vi "Cluster to Element Details.vi"(8 "error in":errorcluster, 11 "Cluster":variant) -> (0 "error out":errorcluster, 1 "gRPC Enum Metadata":T1[](array[typedef]), 2 "More Cluster":variant[](array[variant]), 3 "gRPC Message Metadata":T2)   [LabVIEW 2019, in "grpc-lvsupport.lvlib"]
uses:
  grpc-lvsupport.lvlib
  typeDefs/Message Metadata.ctl
  typeDefs/Message Element Metadata.ctl
  typeDefs/Message Element Type.ctl
  typeDefs/Enum Metadata.ctl
  <vilib>/Utility/Data Type/NI_Data Type.lvlib
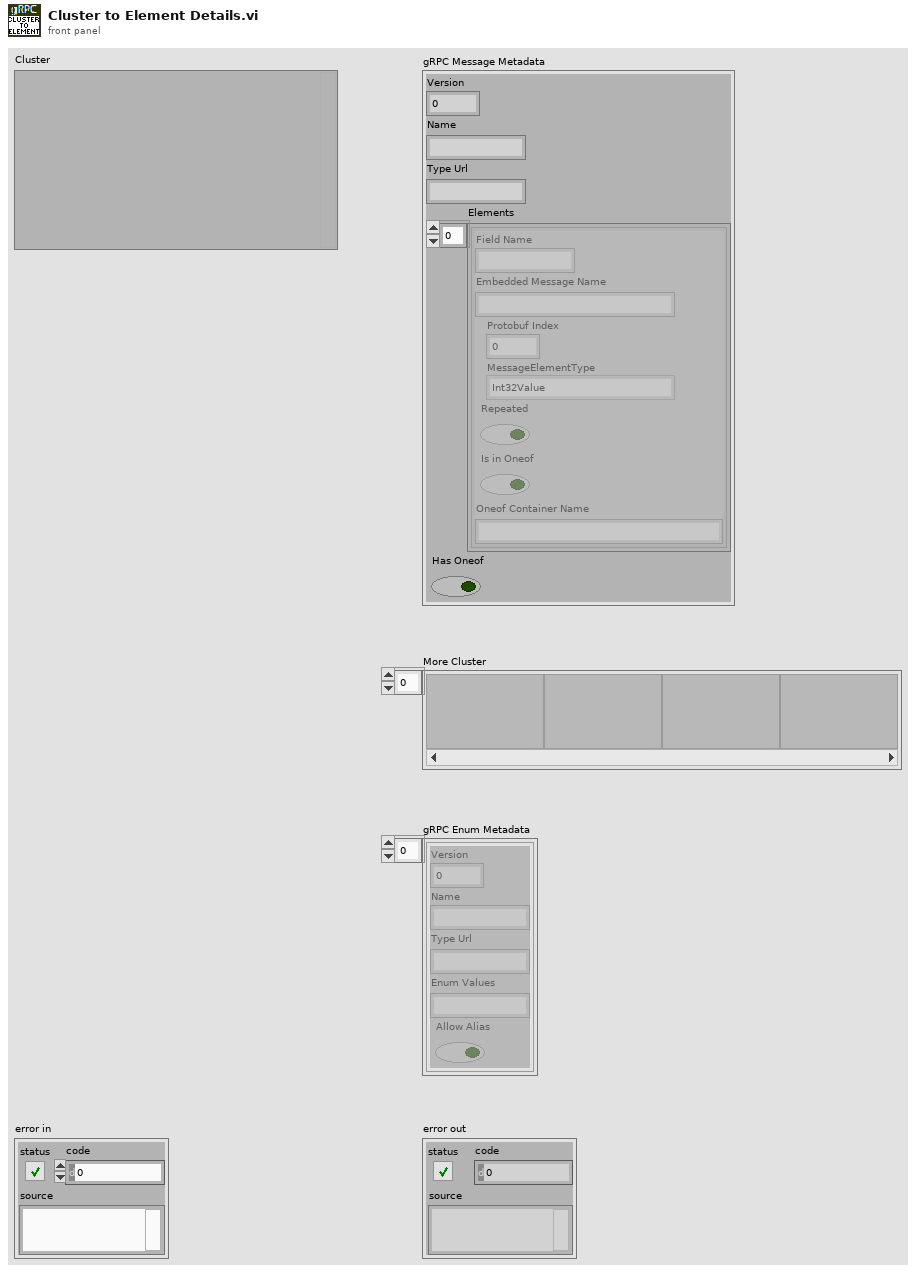
[diagram p1: front panel]
types:
  T1 = typedef "grpc-lvsupport.lvlib/Enum Metadata.ctl" = cluster{"Version":i32, "Name":string, "Type Url":string, "Enum Values":string, "Allow Alias":bool}
  T2 = typedef "grpc-lvsupport.lvlib/Message Metadata.ctl" = cluster{"Version":i32, "Name":string, "Type Url":string, "Elements":T3[], "Has Oneof":bool}
  T3 = typedef "grpc-lvsupport.lvlib/Message Element Metadata.ctl" = cluster{"Field Name":string, "Embedded Message Name":string, "Protobuf Index":i32, "MessageElementType":T4, "Repeated":bool, "Is in Oneof":bool, "Oneof Container Name":string}
  T4 = typedef "grpc-lvsupport.lvlib/Message Element Type.ctl" = enum32{"Int32Value", "FloatValue", "DoubleValue", "BoolValue", "StringValue", "MessageValue", "Int64Value", "UInt32Value", "UInt64Value", "EnumValue", "Bytes", "Fixed64", "Fixed32", "SFixed64", "SFixed32", "SInt64", "SInt32"}
  T5 = typedef "NI_Data Type.lvlib/Data Type.ctl" = enum8{"Invalid Type", "Void", "I8", "I16", "I32", "I64", "U8", "U16", "U32", "U64", "Single Float", "Double Float", "Extended Float", "Single Complex", "Double Complex", "Extended Complex", "Enum U8", "Enum U16", "Enum U32", "Enum U64", "Single Float With Unit", "Double Float With Unit", "Extended Float With Unit", "Single Complex with Unit", "Double Complex with Unit", "Extended Complex with Unit", "Boolean", "String", "Path", "Picture", "Tag", "Array", "Cluster", "Variant", "LV Variant", "Waveform", "Timestamp", "Digital Waveform", "Digital Data", "ExpressData", "Refnum", "External Data", "VI", "Poly VI", "LabVIEW Class Instance", "Fixed Point", "Set Collection", "Map Collection"}
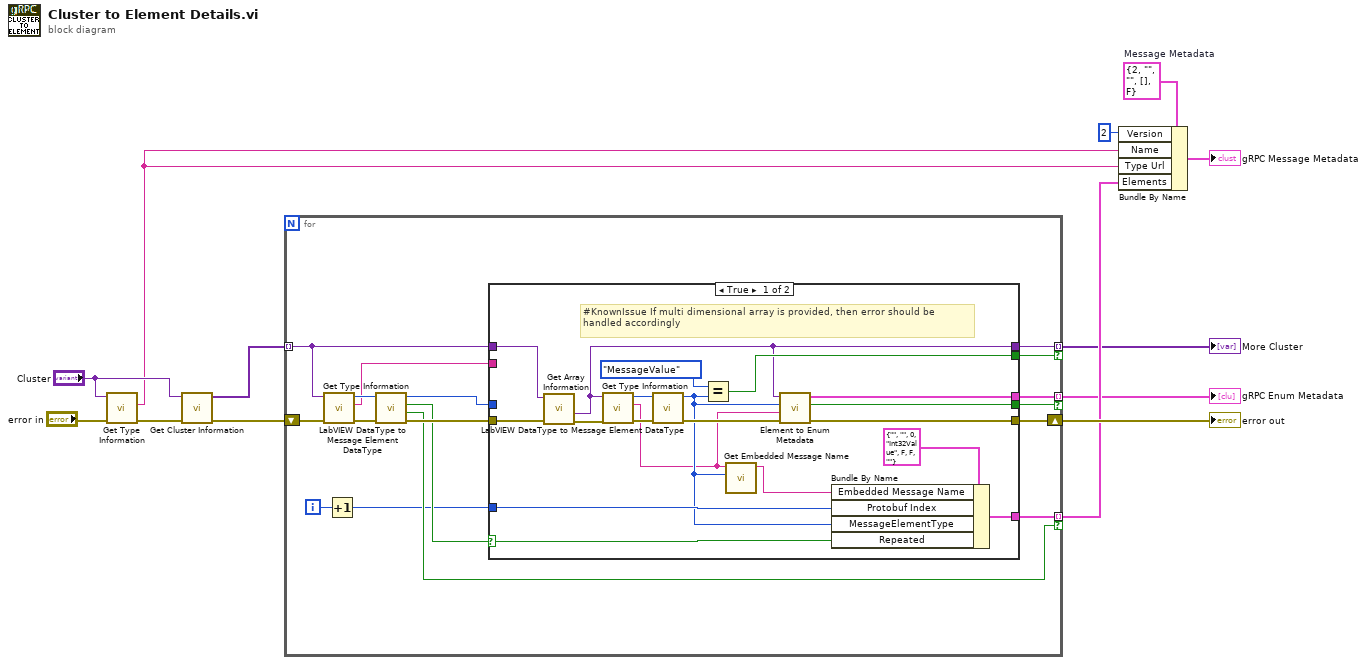
[diagram p0: block diagram]
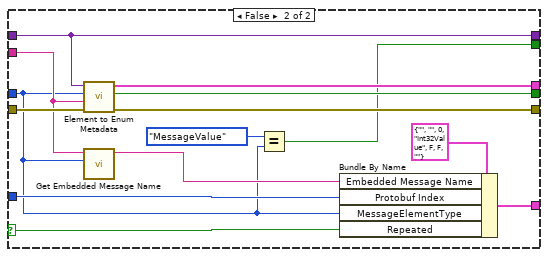
[diagram p2: hidden frame]
diagram:
  w9 = T2 {"Version"=2, "Name"="", "Type Url"="", "Elements"=[], "Has Oneof"=FALSE}  # Message Metadata
  n1 = call <vilib>:"Get Type Information.vi"("error in (no error)"="error in", "variant"="Cluster") -> ("error out"=w13:errorcluster, "name"=w5:string)  [unwired: 5 in, 3 out]
  n2 = call <vilib>:"Get Cluster Information.vi"("error in (no error)"=w13, "variant"="Cluster") -> ("error out"=w12:errorcluster, "cluster elements"=w6:variant[])  [unwired: 8 in]
  n3 = for {
    tunnel: w6 -> [w21] mode=indexing
    tunnel: [w23] -> w4 mode=indexing if=w22
    shift-right: [w27] -> w11
    shift-left: w12 -> [w30]
    tunnel: [w18] -> w3 mode=indexing if=w17
    tunnel: [w15] -> w1 mode=indexing if=w14
    i -> [w26]
    n4 = call <vilib>:"Get Type Information.vi"("error in (no error)"=w30, "variant"=w21) -> ("error out"=w29:errorcluster, "name"=w19:string, "type"=w25:T5)  [unwired: 5 in, 2 out]
    n5 = Increment(x=w26) -> (x+1=w20:i32)
    n6 = call "LabVIEW DataType to Message Element DataType.vi"("error in"=w29, "type"=w25) -> ("error out"=w28:errorcluster, "Supported?"=w22:bool, "Array?"=w24:bool, "MessageElementType"=w16:T4)  [unwired: 6 in]
    n7 = case shown="True" w24 {
      selector: w24 -> [w44 w61]
      tunnel: w20 -> [w46 w63]
      tunnel: [w43 w60] -> w23
      tunnel: w28 -> [w49 w59]
      tunnel: w21 -> [w42 w58]
      tunnel: [w36 w57] -> w27
      tunnel: w19 -> [_ w54]
      tunnel: [w33 w58] -> w18
      tunnel: [w39 w50] -> w17
      tunnel: w16 -> [_ w52]
      tunnel: [w34 w56] -> w15
      tunnel: [w35 w55] -> w14
      frame True {
        # "#KnownIssue If multi dimensional array is provided, then error should be handled accordingly"
        n8 = call <vilib>:"Get Array Information.vi"("error in (no error)"=w49, "variant"=w42) -> ("error out"=w48:errorcluster, "array element data type"=w33:variant)  [unwired: 6 in, 2 out]
        n9 = call <vilib>:"Get Type Information.vi"("error in (no error)"=w48, "variant"=w33) -> ("error out"=w47:errorcluster, "name"=w31:string, "type"=w41:T5)  [unwired: 5 in, 2 out]
        n10 = call "LabVIEW DataType to Message Element DataType.vi"("error in"=w47, "type"=w41) -> ("error out"=w37:errorcluster, "MessageElementType"=w32:T4)  [unwired: 6 in, 2 out]
        n11 = Equal?(x=Message_Element_Type."MessageValue", y=w32) -> (x = y?=w39:bool)
        n12 = call "Get Embedded Message Name.vi"("MessageElementType"=w32, "Element Name"=w31) -> ("Embedded Message Name"=w38:string)  [unwired: 9 in]
        n13 = call "Element to Enum Metadata.vi"("error in (no error)"=w37, "Name"=w31, "MessageElementType"=w32, "Element"=w33) -> ("error out"=w36:errorcluster, "Is Enum?"=w35:bool, "Enum Metadata"=w34:T1)  [unwired: 5 in]
        n14 = Bundle By Name(cluster=T3 {"Field Name"="", "Embedded Message Name"="", "Protobuf Index"=0, "MessageElementType"=enum."Int32Value", "Repeated"=FALSE, "Is in Oneof"=FALSE, "Oneof Container Name"=""} ("MessageElementMetadata"), "Embedded Message Name"=w38, "Protobuf Index"=w46, "MessageElementType"=w32, "Repeated"=w44) -> (w43:T3)
      }
      frame False {
        n15 = call "Element to Enum Metadata.vi"("error in (no error)"=w59, "Name"=w54, "MessageElementType"=w52, "Element"=w58) -> ("error out"=w57:errorcluster, "Is Enum?"=w55:bool, "Enum Metadata"=w56:T1)  [unwired: 5 in]
        n16 = call "Get Embedded Message Name.vi"("MessageElementType"=w52, "Element Name"=w54) -> ("Embedded Message Name"=w53:string)  [unwired: 9 in]
        n17 = Equal?(x=Message_Element_Type."MessageValue", y=w52) -> (x = y?=w50:bool)
        n18 = Bundle By Name(cluster=T3 {"Field Name"="", "Embedded Message Name"="", "Protobuf Index"=0, "MessageElementType"=enum."Int32Value", "Repeated"=FALSE, "Is in Oneof"=FALSE, "Oneof Container Name"=""} ("MessageElementMetadata"), "Embedded Message Name"=w53, "Protobuf Index"=w63, "MessageElementType"=w52, "Repeated"=w61) -> (w60:T3)
      }
    }
  }
  "More Cluster" <- w3
  "error out" <- w11
  "gRPC Enum Metadata" <- w1
  n19 = Bundle By Name(cluster=w9, "Version"=2, "Name"=w5, "Type Url"=w5, "Elements"=w4) -> (→"gRPC Message Metadata":T2)
